vi "Read External Device States and Message Table Index.vi"(8 "error in (no error)":errorcluster, 11 "Lotis in":refnum<class "PL Lotis TII LS.lvclass">) -> (0 "error out":errorcluster, 1 "message table index":u8, 2 "external device states":u8[](array[numeric]) format="%x", 3 "Lotis out":refnum<class "PL Lotis TII LS.lvclass">)   [LabVIEW 2015, in "PL Lotis TII LS.lvclass"]
doc: "Reads external device states and message table index."
uses:
  PL Lotis TII LS.lvclass
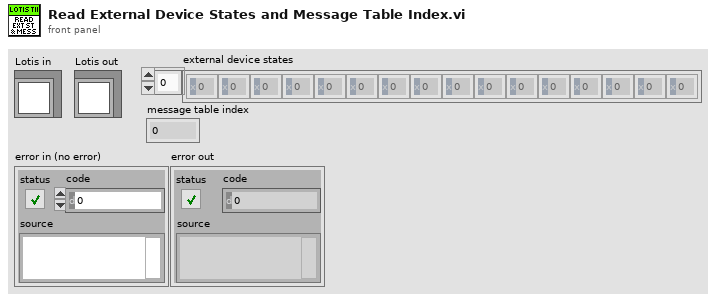
[diagram p1: front panel]
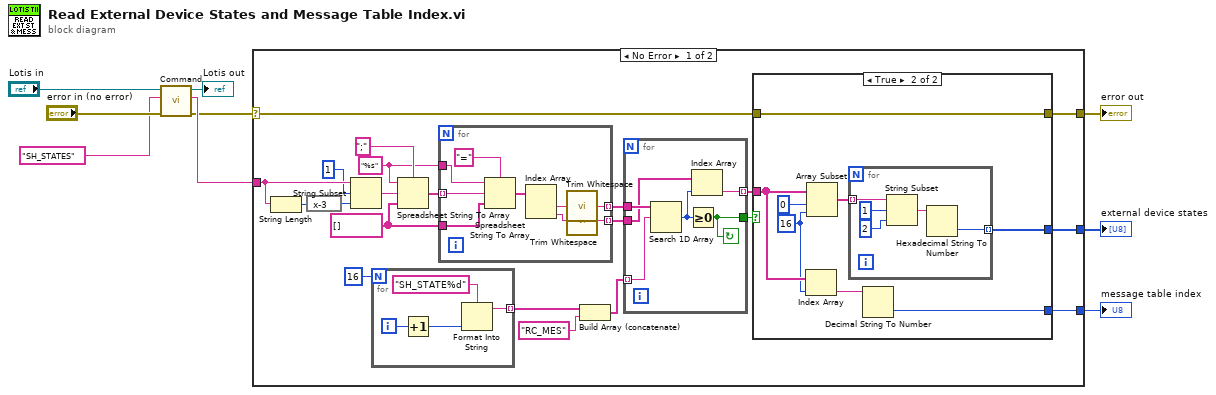
[diagram p0: block diagram]
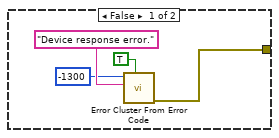
[diagram p2: hidden frame]
diagram:
  n1 = call "Command.vi"("error in (no error)"="error in (no error)", "command"="SH_STATES", "Lotis in"="Lotis in") -> ("error out"=w4:errorcluster, "response data"=w5:string, "Lotis out"=→"Lotis out":refnum<class "PL Lotis TII LS.lvclass">)  [unwired: 6 in]
  n2 = case shown="No Error" w4 {
    selector: w4 -> [w20 w67]
    tunnel: w5 -> [w30 _]
    tunnel: [w19 w67] -> w3
    tunnel: [w11 _] -> w2
    tunnel: [w10 _] -> w1
    frame No Error {
      w23 = "%s" ("format string")
      w22 = string[] [] ("array type (2D Dbl)")
      n3 = String Length(string=w30) -> (length=w28:i32)
      n4 = expression code="x-3"(w28) -> (w27:i32)
      n5 = String Subset(string=w30, offset (0)=1, length (rest)=w27) -> (substring=w26:string)
      n6 = for {
        N: 16 -> [_]
        tunnel: [w31] -> w14 mode=indexing
        i -> [w33]
        n7 = Increment(x=w33) -> (x+1=w32:i32)
        n8 = Format Into String(format string="SH_STATE%d" ("command"), w32) -> (resulting string=w31:string)  [unwired: 2 in, 1 out]
      }
      n9 = Spreadsheet String To Array(delimiter (Tab)=";", format string=w23, spreadsheet string=w26, array type (2D Dbl)=w22) -> (array=w24:string[])
      n10 = for {
        tunnel: w24 -> [w63] mode=indexing
        tunnel: w23 -> [w66]
        tunnel: w22 -> [w64]
        tunnel: [w59] -> w21 mode=indexing
        tunnel: [w58] -> w17 mode=indexing
        n11 = Spreadsheet String To Array(delimiter (Tab)="=", format string=w66, spreadsheet string=w63, array type (2D Dbl)=w64) -> (array=w62:string[])
        n12 = Index Array(array=w62) -> (element #1=w61:string, element #2=w60:string)  [unwired: 2 in]
        n13 = call <vilib>:"Trim Whitespace.vi"("string"=w61) -> ("trimmed string"=w59:string)  [unwired: 1 in]
        n14 = call <vilib>:"Trim Whitespace.vi"("string"=w60) -> ("trimmed string"=w58:string)  [unwired: 1 in]
      }
      n15 = Build Array (concatenate)(w14, "RC_MES") -> (w13:string[])
      n16 = for {
        tunnel: w21 -> [w57]
        tunnel: w13 -> [w56] mode=indexing
        tunnel: [w55] -> w18
        tunnel: w17 -> [w54]
        tunnel: [w52] -> w16 mode=indexing
        stop <- w55 continue-if-true
        n17 = Search 1D Array(1D array=w57, element=w56) -> (index of element=w53:i32)  [unwired: 1 in]
        n18 = Greater Or Equal To 0?(x=w53) -> (x >= 0?=w55:bool)
        n19 = Index Array(array=w54, index=w53) -> (element=w52:string)
      }
      n20 = case shown="True" w18 {
        tunnel: w20 -> [_ w46]
        tunnel: [w35 w46] -> w19
        tunnel: w16 -> [_ w42]
        tunnel: [_ w43] -> w11
        tunnel: [_ w39] -> w10
        frame False {
          n21 = call <vilib>:"Error Cluster From Error Code.vi"("show call chain? (False)"=TRUE, "error message (\"\")"="Device response error." ("format string"), "error code (0)"=-1300) -> ("error out"=w35:errorcluster)  [unwired: 6 in]
        }
        frame True {
          w41 = 16 ("length")
          n22 = Index Array(array=w42, index=w41) -> (element=w40:string)
          n23 = Array Subset(array=w42, index=0, length=w41) -> (w44:string[])
          n24 = for {
            tunnel: w44 -> [w48] mode=indexing
            tunnel: [w47] -> w43 mode=indexing
            n25 = String Subset(string=w48, offset (0)=1, length (rest)=2 ("length (rest)")) -> (substring=w50:string)
            n26 = Hexadecimal String To Number(string=w50) -> (number=w47:u32)  [unwired: 2 in, 1 out]
          }
          n27 = Decimal String To Number(string=w40) -> (number=w39:i32)  [unwired: 2 in, 1 out]
        }
      }
    }
    frame Error {
    }
  }
  "error out" <- w3
  "external device states" <- w2
  "message table index" <- w1
